vi "Average Waveforms.vi"(1 "N-Sample Waveforms":waveform(dbl)[](array[waveform])) -> (0 "1-Sample Average Waveforms":waveform(dbl)[](array[waveform]))   [LabVIEW 2021, in "Acquisition.lvlib"]
doc: "Take the average of the samples in each waveform and return them as one-sample waveforms."
uses:
  Acquisition.lvlib
  <vilib>/Analysis/baseanly.llb/Mean (DBL).vi
  <vilib>/Analysis/NI_AALBase.lvlib
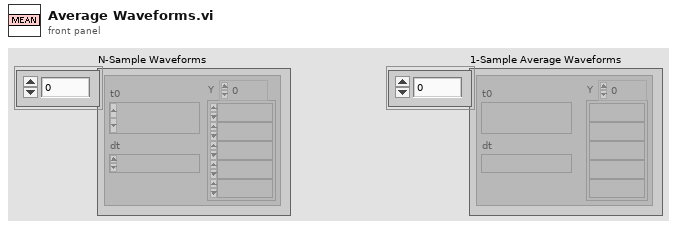
[diagram p1: front panel]
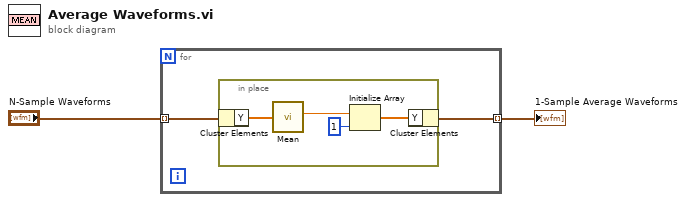
[diagram p0: block diagram]
diagram:
  n1 = for {
    tunnel: "N-Sample Waveforms" -> [w4] mode=indexing
    tunnel: [w3] -> w1 mode=indexing
    n2 = in-place {
      n3 = in-place-cluster #1(w4) -> ("Y"=w8:dbl[])
      n4 = call-poly <vilib>:"Mean.vi"("X"=w8) -> ("mean"=w6:dbl)  [unwired: 1 out]
      n5 = Initialize Array(w6, 1 ("dimension size")) -> (w5:dbl[])
      n6 = in-place-cluster #1("Y"=w5) -> (w3:waveform(dbl))
    }
  }
  "1-Sample Average Waveforms" <- w1
